vi "Update Input Polarity.vi"   [LabVIEW 2014, in "SLSC configuration Shared.lvlib"]
doc: "Sets the input polarity of the pins on the chip."
uses:
  SLSC configuration Shared.lvlib
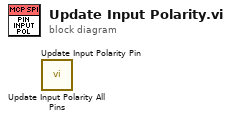
[diagram p0: block diagram]
diagram:
  n1 = call "Update Input Polarity All Pins.vi"() -> ()  [unwired: 9 in, 3 out]
  n2 = call "Update Input Polarity Pin.vi"() -> ()  [unwired: 9 in, 3 out]
